vi "ad get dev info.vi"(8 "error in (no error)":errorcluster, 10 "info":T1, 11 "adh":i32) -> (0 "error out":errorcluster, 2 "info out":T1, 3 "function return":i32)   [LabVIEW 2021, in "libad4.lvlib"]
doc: "LIBAD4 function: ad_get_dev_info (int32_t adh, struct ad_device_info *info);\n\nReturns infromation about the device associated with the passed device handle `adh`."
uses:
  <userlib>/libad4/libad4.lvlib
  <userlib>/libad4/libad4.dll
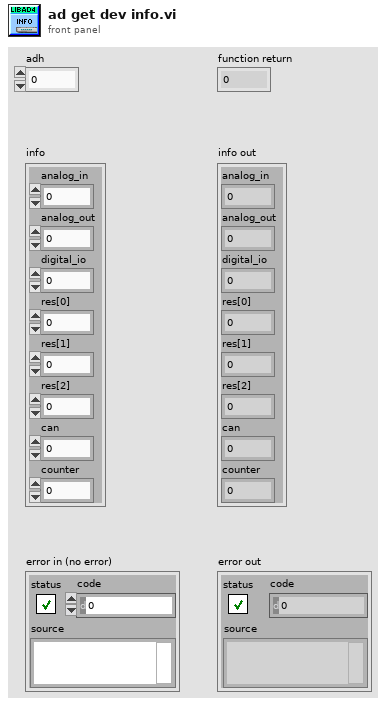
[diagram p1: front panel]
types:
  T1 = cluster{"analog_in":i32, "analog_out":i32, "digital_io":i32, "res[0]":i32, "res[1]":i32, "res[2]":i32, "can":i32, "counter":i32}
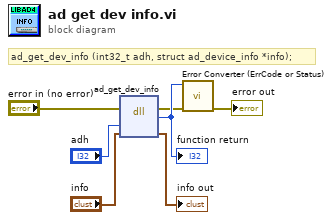
[diagram p0: block diagram]
diagram:
  # "ad_get_dev_info (int32_t adh, struct ad_device_info *info);"
  n1 = dll-call lib="C:/Program Files/National Instruments/LabVIEW 2021/user.lib/libad4/libad4.*" fn="ad_get_dev_info"(error in="error in (no error)", "adh"="adh", "info"="info") -> (error out=w2:errorcluster, w7:i32, "info"=→"info out":T1)  [unwired: 3 in, 1 out]
  "function return" <- w7
  n2 = call <userlib>:"Error Converter (ErrCode or Status).vi"("error in (no error)"=w2, "error code"=w7) -> ("error out"=→"error out":errorcluster)  [unwired: 9 in]
